vi "Enqueue many states to model loop.vi"(8 "error in (no error)":errorcluster, 9 "Following state if error":string, 10 "Enqueued data":variant[](array[variant]), 11 "Enqueued states":string) -> (0 "error out":errorcluster, 2 "Number of states enqueued":i32, 3 "States enqueued":string[](array[string]))   [LabVIEW 2018]
doc: "Enqueued States: Case-insensitive strings that names the cases, one per line, that these entries in the queue will run. Blank lines will be discarded, and will NOT be matched to Variant data inputs.\nEnqueued Data: Variants containing any data needed by the case in the queue. Should match 1:1 to multiple lines in the \"Enqueued States\" input, but if it's longer or shorter than the number of lines it will be either trimmed or extended with null values, as needed.\n\nOptional input:\nFollowing state if error: If left blank, any error in the model loop will clear the model queue and send the error as data to the default \"Error Handler\" state. If filled in, instead of going to the error state next it will go to the specified state, with the error enqueued as the \"Data\" variant. If different following states are needed, use multiple \"Enqueue 1 state\" VIs instead of this single VI."
uses:
  Model queue data.ctl
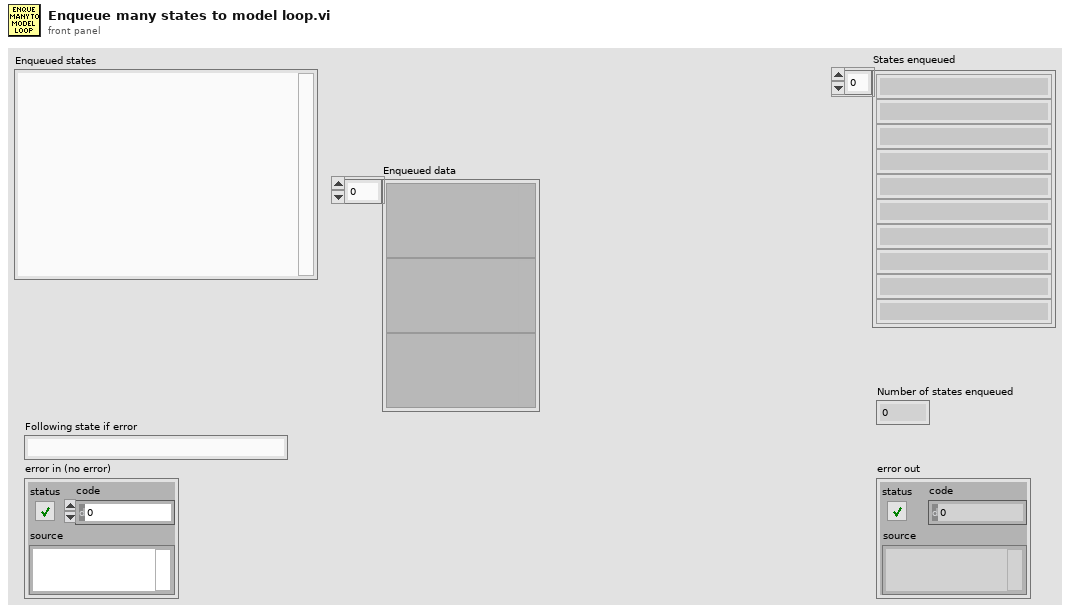
[diagram p1: front panel]
types:
  T1 = typedef "Model queue data.ctl" = cluster{"State":string, "Data":variant, "Next state if error":string}
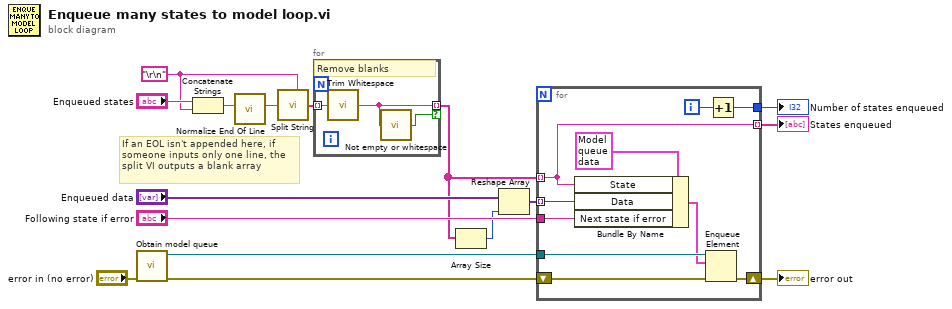
[diagram p0: block diagram]
diagram:
  w4 = "\r\n"
  # "If an EOL isn't appended here, if someone inputs only one line, the split VI outputs a blank array"
  n1 = call "Obtain model queue.vi"("error in (no error)"="error in (no error)") -> ("error out"=w15:errorcluster, "Model loop queue"=w14:refnum<queue>)  [unwired: 9 in]
  n2 = Concatenate Strings("Enqueued states", w4) -> (w5:string)
  n3 = call <vilib>:"Normalize End Of Line.vi"("string in"=w5) -> ("string out"=w3:string)  [unwired: 7 in]
  n4 = call <vilib>:"Split String.vi"("Split Pattern"=w4, "Input String"=w3) -> ("Split String"=w8:string[])  [unwired: 5 in]
  n5 = for {
    tunnel: w8 -> [w19] mode=indexing
    tunnel: [w18] -> w7 mode=indexing if=w17
    # "Remove blanks"
    n6 = call <vilib>:"Trim Whitespace.vi"("string"=w19) -> ("trimmed string"=w18:string)  [unwired: 1 in]
    n7 = call <userlib>:"Not empty or whitespace.vi"("String"=w18) -> ("Not empty or all whitespace"=w17:bool)  [unwired: 4 in]
  }
  n8 = Array Size(array=w7) -> (size(s)=w10:i32)
  n9 = Reshape Array("Enqueued data", w10) -> (w9:variant[])
  n10 = for {
    tunnel: w14 -> [w28]
    tunnel: "Following state if error" -> [w24]
    shift-right: [w25] -> w13
    shift-left: w15 -> [w29]
    tunnel: w9 -> [w23] mode=indexing
    tunnel: w7 -> [w22] mode=indexing
    tunnel: [w22] -> w2 mode=indexing
    tunnel: [w20] -> w1
    i -> [w21]
    n11 = Bundle By Name(cluster=T1 {"State"="", "Data"=variant, "Next state if error"=""} ("element"), "State"=w22, "Data"=w23, "Next state if error"=w24) -> (w26:T1)
    n12 = Enqueue Element(queue=w28, element=w26, error in (no error)=w29) -> (error out=w25:errorcluster)  [unwired: 1 in, 2 out]
    n13 = Increment(x=w21) -> (x+1=w20:i32)
  }
  "error out" <- w13
  "States enqueued" <- w2
  "Number of states enqueued" <- w1
